vi "formas.vi"(8 "error in (no error)":errorcluster, 11 "Image Src":T1) -> (0 "error out":errorcluster, 3 "Classes (Particle Classification 1)":string[](array[string]))   [LabVIEW 2020, in "Analisis.lvlib"]
uses:
  Analisis.lvlib
  <vilib>/vision/Image Controls.llb/IMAQ Image.ctl
  <vilib>/vision/Classification.llb/IMAQ Classifier Read Options.ctl
  <vilib>/vision/NI_Vision_Development_Module.lvlib
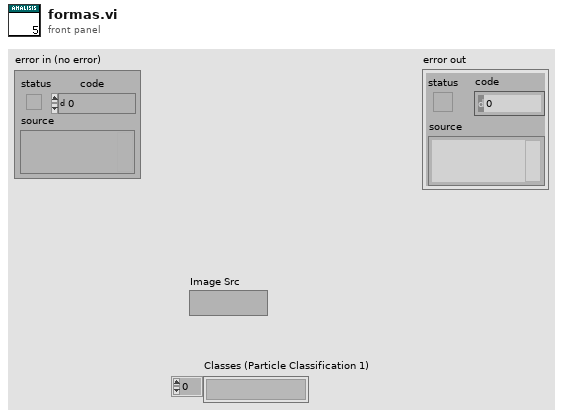
[diagram p1: front panel]
types:
  T1 = typedef "IMAQ Image.ctl" = refnum<image>
  T2 = cluster{"Preprocessing Options":cluster{"Method 2":i32, "Looking for":i32, "Threshold Range":cluster{"Lower value":sgl, "Upper value":sgl}, "Threshold Limits":cluster{"Lower value":sgl, "Upper value":sgl}, "Reject Border":bool, "# of Erosions":i32, "Kernel Size":cluster{"Lower value":i32, "Upper value":i32}, "Deviation Factor":dbl}, "Nearest Neighbor Options":cluster{"Method":i32, "Metric":i32, "k":i32}, "Particle Options":cluster{"Scale Dependant":bool, "Scale Factor":sgl, "Symmetry Dependant":bool, "Symmetry Factor":sgl}}
  T3 = cluster{"Global Rectangle":i32[], "Contours":cluster{"ID":enum32{"External", "Internal"}, "Type":u32, "Coordinates":i32[]}[]}
  T4 = cluster{"histogram":u32[], "Minimal Value":sgl, "Maximal Value":sgl, "Starting Value":sgl, "Interval Width":sgl, "Mean Value":sgl, "Standard  Variation":sgl, "Area (pixels)":i32}
  T5 = typedef "Image Type" = u32
  T6 = cluster{"Method 2":i32, "Looking for":i32, "Threshold Range":cluster{"Lower value":sgl, "Upper value":sgl}, "Threshold Limits":cluster{"Lower value":sgl, "Upper value":sgl}, "Reject Border":bool, "# of Erosions":i32, "Kernel Size":cluster{"Lower value":i32, "Upper value":i32}, "Deviation Factor":dbl}
  T7 = typedef "IMAQ Classifier Read Options.ctl" = i32
  T8 = typedef "IMAQ Classifier Session.ctl" = refnum<k1>
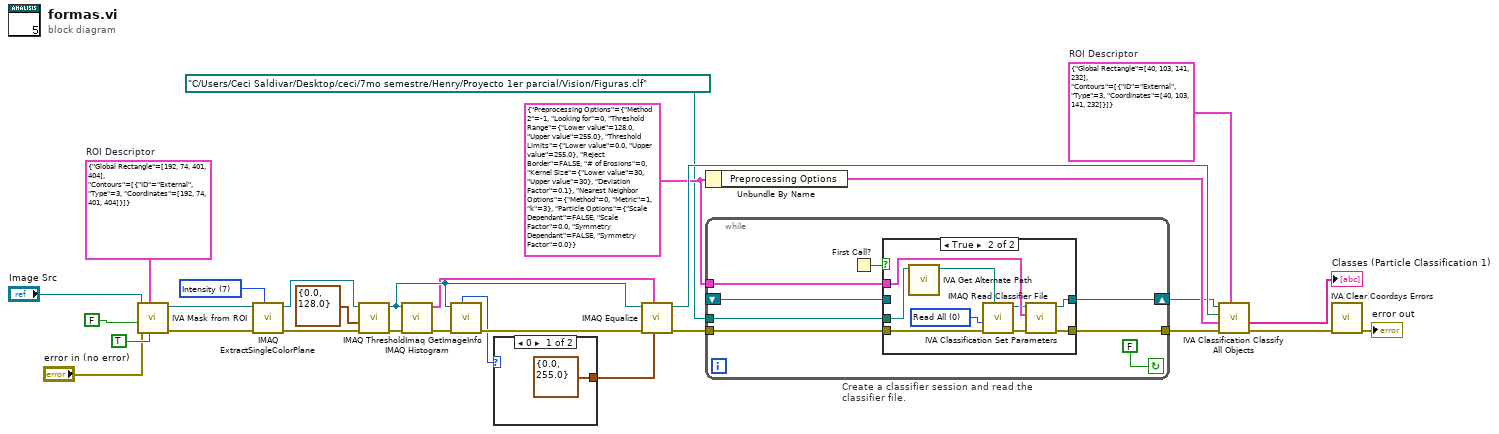
[diagram p0: block diagram]
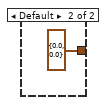
[diagram p3: hidden frame]
diagram:
  w23 = T2 {"Preprocessing Options"={"Method 2"=-1, "Looking for"=0, "Threshold Range"={"Lower value"=128.0, "Upper value"=255.0}, "Threshold Limits"={"Lower value"=0.0, "Upper value"=255.0}, "Reject Border"=FALSE, "# of Erosions"=0, "Kernel Size"={"Lower value"=30, "Upper value"=30}, "Deviation Factor"=0.1}, "Nearest Neighbor Options"={"Method"=0, "Metric"=1, "k"=3}, "Particle Options"={"Scale Dependant"=FALSE, "Scale Factor"=0.0, "Symmetry Dependant"=FALSE, "Symmetry Factor"=0.0}} ("Parameters")
  w24 = T3 {"Global Rectangle"=[40, 103, 141, 232], "Contours"=[{"ID"=enum."External", "Type"=3, "Coordinates"=[40, 103, 141, 232]}]}  # ROI Descriptor
  w8 = 7 items=["Red", "Green", "Blue", "Hue", "Saturation", "Luminance", "Value", "Intensity"] ("Color Plane")
  w4 = T3 {"Global Rectangle"=[192, 74, 401, 404], "Contours"=[{"ID"=enum."External", "Type"=3, "Coordinates"=[192, 74, 401, 404]}]}  # ROI Descriptor
  n1 = call <vilib>:"IVA Mask from ROI.vi"("Shrink"=TRUE, "ROI Descriptor"=w4, "error in (no error)"="error in (no error)", "Out / In"=FALSE, "Image Src"="Image Src") -> ("error out"=w7:errorcluster, "Image Out"=w9:T1)  [unwired: 5 out]
  n2 = call "IMAQ ExtractSingleColorPlane"("Color Plane"=w8, "error in (no error)"=w7, "Image Src"=w9) -> ("error out"=w10:errorcluster, "Image Dst Out"=w12:T1)  [unwired: 1 in, 6 out]
  n3 = call "IMAQ Threshold"("error in (no error)"=w10, "Range"=cluster{"Lower value":sgl, "Upper value":sgl} {"Lower value"=0.0, "Upper value"=128.0}, "Image Src"=w12) -> ("error out"=w13:errorcluster, "Image Dst Out"=w17:T1)  [unwired: 3 in, 4 out]
  n4 = call "IMAQ Histogram"("error in (no error)"=w13, "Image"=w17) -> ("error out"=w18:errorcluster, "Histogram Report"=w15:T4)  [unwired: 3 in, 5 out]
  n5 = call "Imaq GetImageInfo"("error in (no error)"=w18, "Image"=w17) -> ("error out"=w19:errorcluster, "Image Type"=w16:T5)  [unwired: 8 out]
  n6 = case shown="0" w16 {
    tunnel: [cluster{"Minimum":sgl, "Maximum":sgl} {"Minimum"=0.0, "Maximum"=255.0} ("Range") cluster{"Minimum":sgl, "Maximum":sgl} {"Minimum"=0.0, "Maximum"=0.0} ("Range")] -> w20
    frame 0 {
    }
    frame Default {
    }
  }
  n7 = call "IMAQ Equalize"("Range"=w20, "Histogram Report"=w15, "error in (no error)"=w19, "Image Src"=w17) -> ("error out"=w14:errorcluster, "Image Dst Out"=w29:T1)  [unwired: 2 in, 4 out]
  n8 = Unbundle By Name(w23) -> ("Preprocessing Options"=w27:T6)
  n9 = while "Create a classifier session and read the classifier file." {
    shift-right: [w38] -> w25
    shift-left: _ -> [w37]
    tunnel: w14 -> [w35]
    tunnel: [w34] -> w26
    tunnel: path "C:/Users/Ceci Saldivar/Desktop/ceci/7mo semestre/Henry/Proyecto 1er parcial/Vision/Figuras.clf" ("File Path") -> [w33]
    tunnel: w23 -> [w32]
    stop <- FALSE continue-if-true
    n10 = First Call?() -> (First Call?: T/F=w39:bool)
    n11 = case shown="True" w39 {
      tunnel: [w41 w46] -> w38
      tunnel: w37 -> [w41 _]
      tunnel: w35 -> [w40 w50]
      tunnel: [w40 w44] -> w34
      tunnel: w33 -> [_ w43]
      tunnel: w32 -> [_ w48]
      frame False {
      }
      frame True {
        w49 = T7 0 items=["Read All", "Add Samples, Do Not Change Options", "Read Options, Do Not Add Samples"] ("Read Options")
        n12 = call <vilib>:"IVA Get Alternate Path.vi"("Path In"=w43) -> ("Path Out"=w42:path)  [unwired: 10 out]
        n13 = call "IMAQ Read Classifier File"("File Path"=w42, "error in (no error)"=w50, "Read Options"=w49) -> ("error out"=w45:errorcluster, "Classifier Session"=w47:T8)  [unwired: 1 in, 6 out]
        n14 = call <vilib>:"IVA Classification Set Parameters.vi"("error in"=w45, "Paramaters"=w48, "Classifier Session In"=w47) -> ("error out"=w44:errorcluster, "Classifier Session Out"=w46:T8)  [unwired: 7 out]
      }
    }
  }
  n15 = call <vilib>:"IVA Classification Classify All Objects.vi"("ROI Descriptor"=w24, "error in (no error)"=w26, "Preprocessing Options"=w27, "Image"=w29, "Classifier Session"=w25) -> ("error out"=w28:errorcluster, "Classes"=→"Classes (Particle Classification 1)":string[])  [unwired: 5 out]
  n16 = call <vilib>:"IVA Clear Coordsys Errors.vi"("error in (no error)"=w28) -> ("error out"=→"error out":errorcluster)  [unwired: 10 in]
